vi "Preview Button States.vi"(10 "Event Registration Refnum":refnum<event-registration>) -> (3 "Preview":picture)   [LabVIEW 2012]
types:
  T1 = typedef "imagedata.ctl" = cluster{"image type":i32, "image depth":i32, "image":u8[], "mask":u8[], "colors":u32[], "Rectangle":cluster{"left":i16, "top":i16, "right":i16, "bottom":i16}}
  T2 = cluster{"left":i16, "top":i16, "right":i16, "bottom":i16}
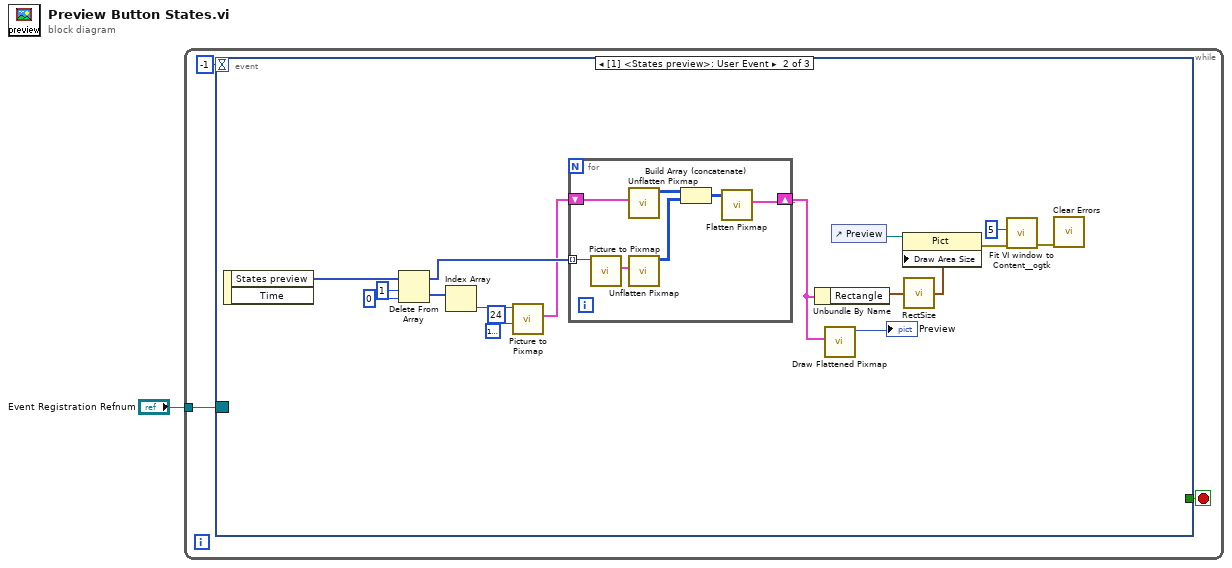
[diagram p0: block diagram]
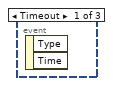
[diagram p2: hidden frame]
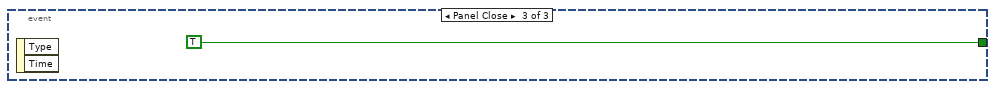
[diagram p3: hidden frame]
diagram:
  n1 = while {
    tunnel: "Event Registration Refnum" -> [w3]
    stop <- w2 stop-if-true
    n2 = event shown="[1] <States preview>: User Event" {
      selector: w3 -> [_ _ _]
      dyn-events: _ -> [_ _ _]
      timeout: -1 -> [_ _ _]
      tunnel: [_ _ TRUE] -> w2
      event Timeout {
        n3 = event-data() -> ()  [unwired: 3 out]
      }
      event User Event {
        (unwired) u32 16777216
        n4 = event-data() -> ("States preview"=w10:picture[])  [unwired: 2 out]
        n5 = Delete From Array(array=w10, length=1, index=0) -> (deleted portion=w15:picture[], array with subset deleted=w14:picture[])
        n6 = Index Array(array=w15) -> (element=w19:picture)  [unwired: 1 in]
        n7 = call <vilib>:"Picture to Pixmap.vi"("depth"=24, "picture"=w19) -> ("image data"=w9:T1)  [unwired: 2 in, 7 out]
        n8 = for {
          tunnel: w14 -> [w27] mode=indexing
          shift-right: [w23] -> w13
          shift-left: w9 -> [w22]
          n9 = call <vilib>:"Picture to Pixmap.vi"("picture"=w27) -> ("image data"=w21:T1)  [unwired: 3 in, 7 out]
          n10 = call <vilib>:"Unflatten Pixmap.vi"("image data"=w22) -> ("24-bit pixmap"=w26:u32[][])  [unwired: 10 out]
          n11 = call <vilib>:"Unflatten Pixmap.vi"("image data"=w21) -> ("24-bit pixmap"=w25:u32[][])  [unwired: 10 out]
          n12 = Build Array (concatenate)(w26, w25) -> (w24:u32[][])
          n13 = call <vilib>:"Flatten Pixmap.vi"("24-bit pixmap"=w24) -> ("image data"=w23:T1)  [unwired: 5 in, 5 out]
        }
        n14 = Unbundle By Name(w13) -> ("Rectangle"=w12:T2)
        n15 = call <vilib>:"Draw Flattened Pixmap.vi"("image data"=w13) -> ("new picture"=→"Preview":picture)  [unwired: 1 in, 7 out]
        n16 = control-ref of="Preview"() -> (w5:refnum<vi>)
        n17 = call <vilib>:"RectSize.vi"("rect"=w12) -> ("point"=w11:cluster{"x":i16, "y":i16})
        n18 = property class="Pict"(reference=w5, "Draw Area Size"=w11) -> (error out=w7:errorcluster)  [unwired: 1 in, 1 out]
        n19 = call <userlib>:"Fit VI window to Content__ogtk.vi"("error in (no error)"=w7, "border spacing (2 px)"=5) -> ("error out"=w8:errorcluster)  [unwired: 1 in, 4 out]
        n20 = call <vilib>:"Clear Errors.vi"("error in (no error)"=w8) -> ()  [unwired: 7 out]
      }
      event Panel Close {
        n21 = event-data() -> ()  [unwired: 3 out]
      }
    }
  }
